vi "Input String Validation.vi"(6 "Input Type":T2 caption="Input Type (default: IP)", 7 "Handle NIVS Errors Internally?":bool=TRUE caption="Handle NIVS Errors Internally? (T)", 8 "Error In":errorcluster, 10 "String to check":string="  ", 11 "Item Ref in":T1 format="%.0x") -> (0 "Error Out":errorcluster, 1 "Valid?":bool, 2 "String to check dup":string="  ", 3 "Item Ref out":T1 format="%.0x")   [LabVIEW 2018, in "Vires VTD System Explorer.lvlib"]
uses:
  Vires VTD System Explorer.lvlib
  Shared/Input Validation Type.ctl
  <vilib>/NI Veristand/Custom Device API/Custom Device Item Ref.ctl
  <vilib>/regexp/Match Regular Expression.xnode
  <vilib>/NI Veristand/Custom Device API/Custom Device API.lvlib
  Shared/Vires VTD Shared.lvlib
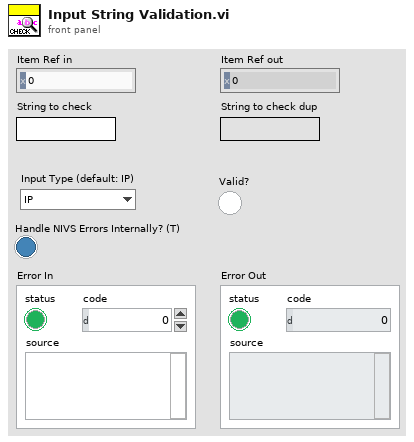
[diagram p1: front panel]
types:
  T1 = typedef "Custom Device API.lvlib/Custom Device Item Ref.ctl" = u64
  T2 = typedef "Vires VTD Shared.lvlib/Input Validation Type.ctl" = enum16{"IP"}
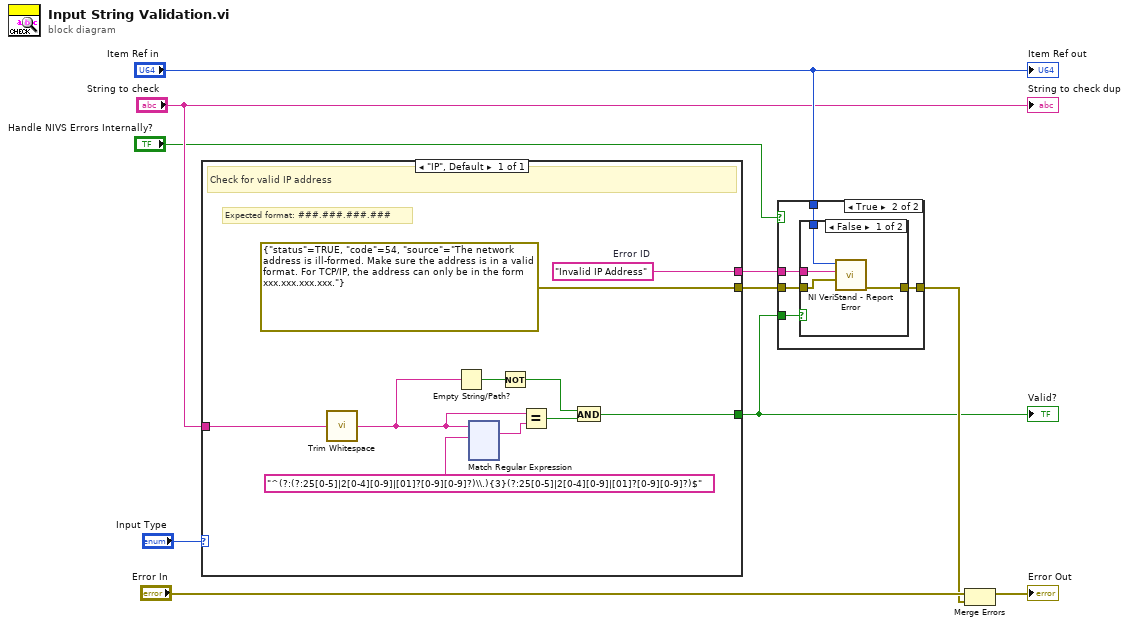
[diagram p0: block diagram]
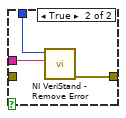
[diagram p3: hidden frame]
diagram:
  n1 = case shown="\"IP\", Default" "Input Type" {
    tunnel: "String to check" -> [w19]
    tunnel: [w16] -> w5
    tunnel: [w12] -> w2
    tunnel: [errorcluster {"status"=TRUE, "code"=54, "source"="The network address is ill-formed. Make sure the address is in a valid format. For TCP/IP, the address can only be in the form xxx.xxx.xxx.xxx."} ("error out")] -> w1
    frame "IP", Default {
      w12 = "Invalid IP Address"  # Error ID
      # "Expected format: ###.###.###.###"
      # "Check for valid IP address"
      n2 = call <vilib>:"Trim Whitespace.vi"("string"=w19) -> ("trimmed string"=w15:string)  [unwired: 1 in]
      n3 = Empty String/Path?(string/path=w15) -> (empty?=w14:bool)
      n4 = xnode "Match Regular Expression"("input string"=w15, "regular expression"="^(?:(?:25[0-5]|2[0-4][0-9]|[01]?[0-9][0-9]?)\\.){3}(?:25[0-5]|2[0-4][0-9]|[01]?[0-9][0-9]?)$") -> ("whole match"=w18:string)  [unwired: 4 in, 4 out]
      n5 = Not(x=w14) -> (.not. x?=w13:bool)
      n6 = Equal?(x=w15, y=w18) -> (x = y?=w17:bool)
      n7 = And(x=w13, y=w17) -> (x .and. y?=w16:bool)
    }
  }
  "Valid?" <- w5
  n8 = case shown="True" "Handle NIVS Errors Internally?" {
    tunnel: [_ w139] -> w7
    tunnel: "Item Ref in" -> [_ w138]
    tunnel: w5 -> [_ w137]
    tunnel: w2 -> [_ w136]
    tunnel: w1 -> [_ w135]
    frame False {
    }
    frame True {
      n9 = case shown="False" w137 {
        tunnel: [w143 w146] -> w139
        tunnel: w138 -> [w142 w145]
        tunnel: w136 -> [w141 w144]
        tunnel: w135 -> [w140 _]
        frame False {
          n10 = call <vilib>:"NI VeriStand - Report Error.vi"("New Error"=w140, "Error ID"=w141, "Node Ref in"=w142) -> ("error out"=w143:errorcluster)  [unwired: 7 in, 1 out]
        }
        frame True {
          n11 = call <vilib>:"NI VeriStand - Remove Error.vi"("Error ID"=w144, "Node Ref in"=w145) -> ("error out"=w146:errorcluster)  [unwired: 8 in, 1 out]
        }
      }
    }
  }
  n12 = Merge Errors("Error In", w7) -> (→"Error Out":errorcluster)
  "String to check dup" <- "String to check"
  "Item Ref out" <- "Item Ref in"
